vi "HighSpeedGrab.vi"(0 "IMAQ Refnum in":refnum<k11>, 1 "Tracking enabled?":bool, 3 "QTrk Instance":T3, 4 "ROIs":cluster{"X":i32, "Y":i32}[](array[cluster]), 6 "stop":refnum<vi>, 7 "Type":T2, 8 "Send to queue?":bool, 9 "#ROI":u32, 10 "Output Queue":refnum<queue>, 12 "ResultManager":T1, 13 "ROI Size":cluster{"X":i32, "Y":i32}) -> (14 "IMAQ Refnum out":refnum<k11>)   [LabVIEW 2011]
uses:
  qtrk/QTrk.llb/QTrkInstance.ctl
  BeadTracker2.llb/CmdEnum_CameraFrameType.ctl
  qtrk/QTrk.llb/ResultManagerInstance.ctl
  BeadTracker2.llb/CmdData_NewFrame.ctl
  <vilib>/vision/Image Controls.llb/IMAQ Image.ctl
  qtrk/QTrk.llb/QTrkDLL.vi
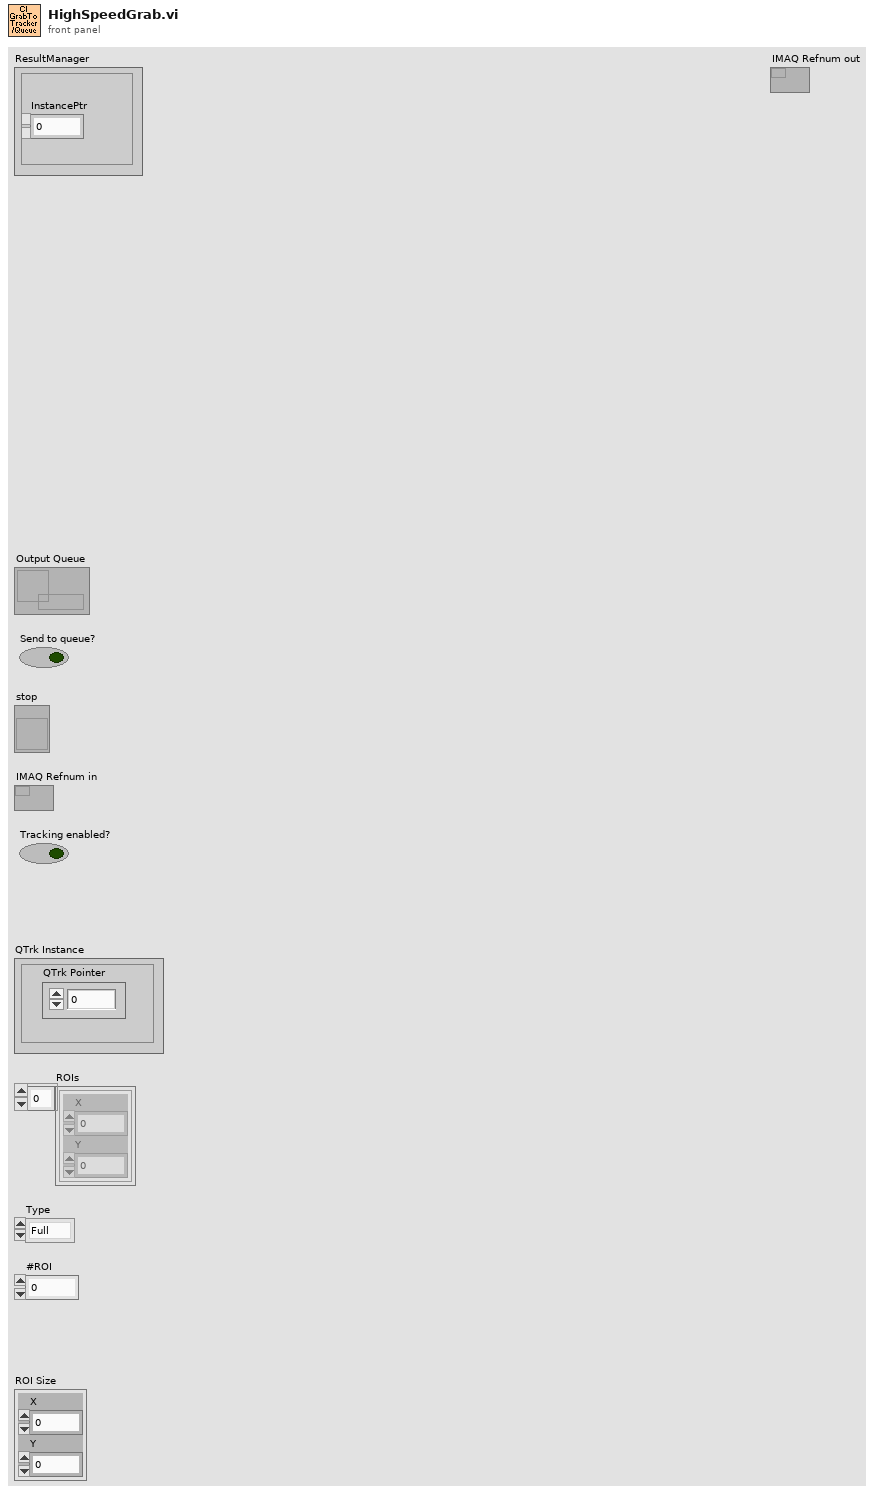
[diagram p1: front panel]
types:
  T1 = typedef "ResultManagerInstance.ctl" = cluster{"InstancePtr":u64}
  T2 = typedef "CmdEnum_CameraFrameType.ctl" = enum16{"Full", "HardwareROI", "EndGrabMarker"}
  T3 = typedef "QTrkInstance.ctl" = cluster{"QTrk Pointer":u64}
  T4 = typedef "IMAQ Image.ctl" = refnum<image>
  T5 = typedef "CmdData_NewFrame.ctl" = cluster{"Buffer Image":T4, "Frame #":i32, "Hardware ROI Index":i32, "Timestamp":dbl, "Type":T2}
  T6 = enum32{"Map Pixel Pointer", "Unmap Pixel Pointer", "Get Pixels Infos"}
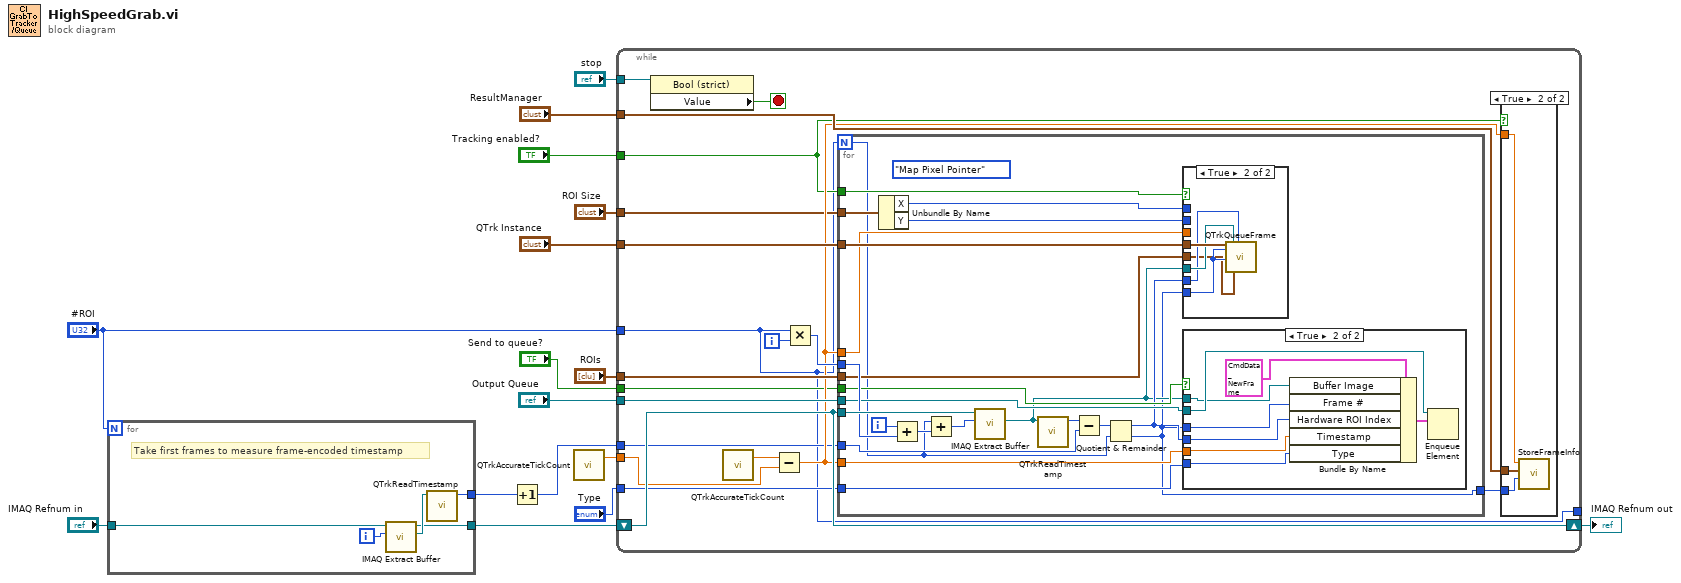
[diagram p0: block diagram]
diagram:
  n1 = for {
    N: "#ROI" -> [_]
    tunnel: "IMAQ Refnum in" -> [w20]
    tunnel: [w19] -> w3
    tunnel: [w17] -> w5
    i -> [w18]
    # "Take first frames to measure frame-encoded timestamp"
    n2 = call <vilib>:"IMAQ Extract Buffer.vi"("Buffer to extract"=w18, "IMAQ Session In"=w20) -> ("Image Out"=w21:T4, "IMAQ Session Out"=w19:refnum<k11>)  [unwired: 4 in, 4 out]
    n3 = call "QTrkReadTimestamp.vi"("Image"=w21) -> ("timestamp"=w17:u32)  [unwired: 10 in]
  }
  n4 = Increment(x=w5) -> (x+1=w2:u32)
  n5 = call "QTrkAccurateTickCount.vi"() -> ("tick count (ms)"=w6:dbl)  [unwired: 2 in, 1 out]
  n6 = while {
    tunnel: "Output Queue" -> [w33]
    shift-right: [w38] -> w8
    shift-left: w3 -> [w38]
    tunnel: "QTrk Instance" -> [w40]
    tunnel: [w22] -> _
    tunnel: w6 -> [w36]
    tunnel: "ROIs" -> [w35]
    tunnel: "ResultManager" -> [w34]
    tunnel: "Type" -> [w30]
    tunnel: "Send to queue?" -> [w29]
    tunnel: w2 -> [w28]
    tunnel: "ROI Size" -> [w27]
    tunnel: "stop" -> [w25]
    tunnel: "Tracking enabled?" -> [w23]
    tunnel: "#ROI" -> [w22]
    i -> [w32]
    stop <- w24 stop-if-true
    n7 = property on="Property Node" class="Bool (strict)"(reference=w25) -> ("Value"=w24:bool)  [unwired: 1 in, 2 out]
    n8 = call "QTrkAccurateTickCount.vi"() -> ("tick count (ms)"=w37:dbl)  [unwired: 2 in, 1 out]
    n9 = Subtract(x=w37, y=w36) -> (x-y=w31:dbl)
    n10 = Multiply(x=w22, y=w32) -> (x*y=w39:u32)
    n11 = for {
      N: w22 -> [w49]
      tunnel: w23 -> [w66]
      tunnel: w40 -> [w65]
      tunnel: w38 -> [w64]
      tunnel: w39 -> [w63]
      tunnel: w31 -> [w62]
      tunnel: w35 -> [w61]
      tunnel: w29 -> [w60]
      tunnel: w33 -> [w59]
      tunnel: w31 -> [w57]
      tunnel: w30 -> [w56]
      tunnel: w28 -> [w52]
      tunnel: w27 -> [w53]
      tunnel: [w44] -> w26
      i -> [w58]
      (unwired) T6."Map Pixel Pointer" ("Function")
      n12 = Unbundle By Name(w53) -> ("X"=w51:i32, "Y"=w50:i32)
      n13 = Add(x=w58, y=w63) -> (x+y=w54:u32)
      n14 = Add(x=w49, y=w54) -> (x+y=w55:u32)
      n15 = call <vilib>:"IMAQ Extract Buffer.vi"("Buffer to extract"=w55, "IMAQ Session In"=w64) -> ("Image Out"=w45:T4)  [unwired: 4 in, 5 out]
      n16 = call "QTrkReadTimestamp.vi"("Image"=w45) -> ("timestamp"=w46:u32)  [unwired: 10 in]
      n17 = Subtract(x=w46, y=w52) -> (x-y=w48:u32)
      n18 = Quotient & Remainder(x=w48, y=w49) -> (x-y*floor(x/y)=w47:u32, floor(x/y)=w44:u32)
      n19 = case shown="True" w66 {
        tunnel: w65 -> [_ w79]
        tunnel: w62 -> [_ _]
        tunnel: w61 -> [_ w75]
        tunnel: w51 -> [_ _]
        tunnel: w50 -> [_ _]
        tunnel: w44 -> [_ w76]
        tunnel: w47 -> [_ w77]
        tunnel: w45 -> [_ w78]
        frame False {
        }
        frame True {
          n20 = call "QTrkQueueFrame.vi"("QTrk Instance"=w79, "frame#"=w76, "timestamp"=w76, "Image"=w78, "ROI Positions (corner-based)"=w75, "ZLUT Index offset (0)"=w77) -> ()  [unwired: 11 in, 3 out]
        }
      }
      n21 = case shown="True" w60 {
        tunnel: w59 -> [_ w74]
        tunnel: w45 -> [_ w72]
        tunnel: w57 -> [_ w71]
        tunnel: w56 -> [_ w70]
        tunnel: w44 -> [_ w68]
        tunnel: w47 -> [_ w67]
        frame False {
        }
        frame True {
          n22 = Bundle By Name(cluster=T5 {"Buffer Image"=refnum, "Frame #"=0, "Hardware ROI Index"=0, "Timestamp"=0.0, "Type"=enum."Full"} ("element"), "Buffer Image"=w72, "Frame #"=w68, "Hardware ROI Index"=w67, "Timestamp"=w71, "Type"=w70) -> (w69:T5)
          n23 = Enqueue Element(queue=w74, element=w69) -> ()  [unwired: 2 in, 3 out]
        }
      }
    }
    n24 = case shown="True" w23 {
      tunnel: w34 -> [_ w43]
      tunnel: w31 -> [_ w42]
      tunnel: w26 -> [_ w41]
      frame False {
      }
      frame True {
        n25 = call "StoreFrameInfo.vi"("frame"=w41, "ResultManager"=w43, "Timestamp"=w42) -> ()  [unwired: 9 in]
      }
    }
  }
  "IMAQ Refnum out" <- w8
